vi "Is Clear.vi"(10 "Direction":T1, 11 "Maze":i32[](array[numeric])) -> (1 "Can Move?":bool, 2 "Direction Out":T1, 3 "Maze":i32[](array[numeric]))   [LabVIEW 2020, in "Rain.lvclass"]
uses:
  Rain.lvclass
  Type Defs/Direction Enum.ctl
  Type Defs/SB Type Defs.lvlib
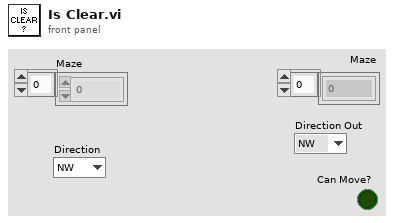
[diagram p1: front panel]
types:
  T1 = typedef "SB Type Defs.lvlib/Direction Enum.ctl" = enum16{"NW", "N", "NE", "E", "SE", "S", "SW", "W"}
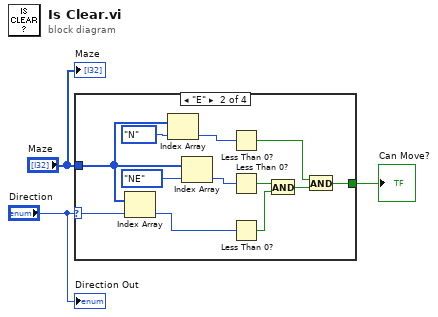
[diagram p0: block diagram]
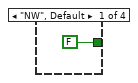
[diagram p2: hidden frame]
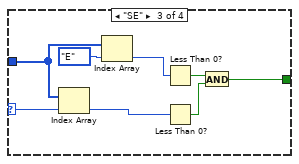
[diagram p3: hidden frame]
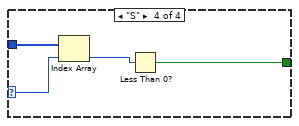
[diagram p4: hidden frame]
diagram:
  n1 = case shown="\"E\"" "Direction" {
    selector: "Direction" -> [_ w15 w23 w28]
    tunnel: "Maze" -> [_ w11 w20 w27]
    tunnel: [FALSE w5 w17 w26] -> w2
    frame "NW", Default {
    }
    frame "E" {
      n2 = Index Array(array=w11, index=w15) -> (element=w16:i32)
      n3 = Index Array(array=w11, index=Direction_Enum."N" ("Direction 2")) -> (element=w10:i32)
      n4 = Index Array(array=w11, index=Direction_Enum."NE" ("Direction 2")) -> (element=w14:i32)
      n5 = Less Than 0?(x=w10) -> (x < 0?=w6:bool)
      n6 = Less Than 0?(x=w14) -> (x < 0?=w8:bool)
      n7 = Less Than 0?(x=w16) -> (x < 0?=w9:bool)
      n8 = And(x=w8, y=w9) -> (x .and. y?=w7:bool)
      n9 = And(x=w6, y=w7) -> (x .and. y?=w5:bool)
    }
    frame "SE" {
      n10 = Index Array(array=w20, index=w23) -> (element=w24:i32)
      n11 = Index Array(array=w20, index=Direction_Enum."E" ("Direction 2")) -> (element=w21:i32)
      n12 = Less Than 0?(x=w21) -> (x < 0?=w18:bool)
      n13 = Less Than 0?(x=w24) -> (x < 0?=w19:bool)
      n14 = And(x=w18, y=w19) -> (x .and. y?=w17:bool)
    }
    frame "S" {
      n15 = Index Array(array=w27, index=w28) -> (element=w25:i32)
      n16 = Less Than 0?(x=w25) -> (x < 0?=w26:bool)
    }
  }
  "Can Move?" <- w2
  "Maze" <- "Maze"
  "Direction Out" <- "Direction"
